vi "Send Triggers Setup.vi"(8 "error in (no error)":errorcluster, 11 "FGPA Ref":T1) -> (0 "error out":errorcluster, 3 "FGPA Ref":T1)   [LabVIEW 2013]
uses:
  RIG-SPECIFIC FILES/FPGA Refs/FPGA Ref.ctl
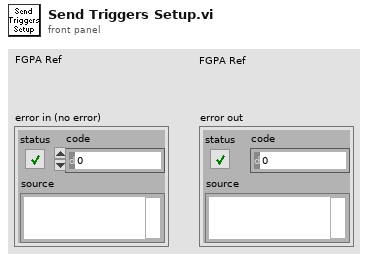
[diagram p1: front panel]
types:
  T1 = typedef "FPGA Ref.ctl" = refnum<k20>
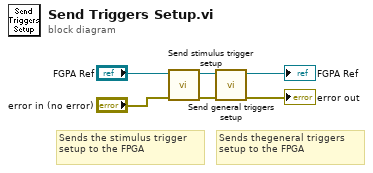
[diagram p0: block diagram]
diagram:
  # "Sends thegeneral triggers setup to the FPGA"
  # "Sends the stimulus trigger setup to the FPGA"
  n1 = call "Send stimulus trigger setup.vi"("error in (no error)"="error in (no error)", "FPGA ref in"="FGPA Ref") -> ("error out"=w4:errorcluster, "FPGA ref out"=w3:T1)  [unwired: 8 in]
  n2 = call "Send general triggers setup.vi"("error in (no error)"=w4, "Refnum in"=w3) -> ("error out"=→"error out":errorcluster, "Refnum out"=→"FGPA Ref":T1)  [unwired: 8 in]
